vi "Multiple Rates Streaming Example.vi"() -> ()   [LabVIEW 2024]
doc: "Streaming multiple channels at different rates to a run."
uses:
  Sift API/Sift Client.lvclass
  Generate Sift Protos/SiftProxy_client/RPC Messages/sift_proxy_v1_ChannelDataType.ctl
  <vilib>/numeric/Random Number (Range) DBL.vi
  Generate Sift Protos/SiftProxy_client/SiftProxy_client.lvlib
  Sift Client.lvlib
panel:
  out "Running":bool
  out "100Hz Channel 3":dbl(knob) scale=0.0..10.0
  out "100Hz Channel 2":dbl(knob) scale=0.0..10.0
  out "100Hz Channel 1":dbl(knob) scale=0.0..10.0
  out "Loop 2 Error":errorcluster
  out "10Hz Channel 3":dbl(knob) scale=0.0..10.0
  out "10Hz Channel 2":dbl(knob) scale=0.0..10.0
  out "10Hz Channel 1":dbl(knob) scale=0.0..10.0
  out "Flush Error":errorcluster
  in  "Stop":bool
  out "Loop 1 Error":errorcluster
  in  "Organization ID":string
  in  "API Key":string
  in  "API URL":string
  # "Multiple Rates Sift Streaming Example"
  # "Instructions\n\n1. Fill in the API URL, API Key, and Organization ID. Visit this URL for more information on authentication\n    https://docs.siftstack.com/docs/api/authentication\n\n2. Start the VI\n\n3. Navigate to the Assets page and open the \"LabVIEW-Example\" asset.\n\n4. You should see the test test channels in the run.\n\n5. Click on the Live button  to see the telemetry update.\n\n6. Click Stop to stop the VI."
  # "This example streams data live from LabVIEW with channels at different rates."
  # "100Hz  Channels"
  # "These values are automatically updated randomly."
  # "Hit this to stop the example."
  # "10Hz  Channels"
  # "These values are automatically updated randomly."
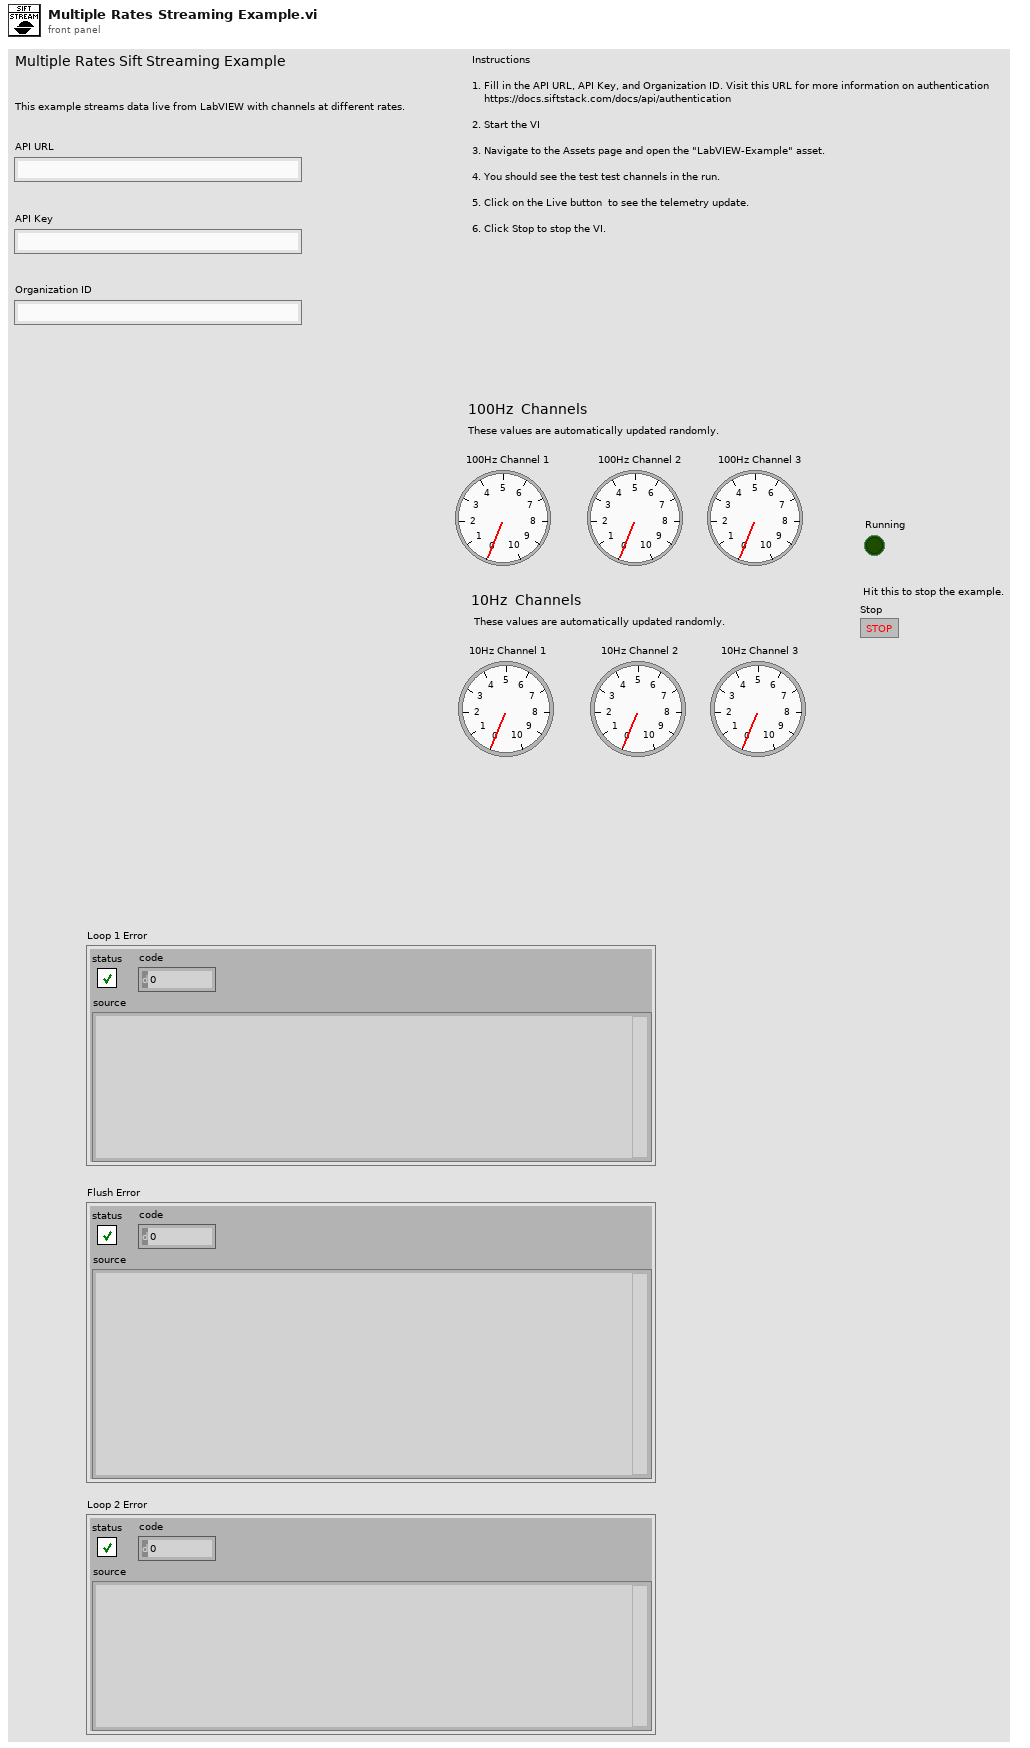
[diagram p1: front panel]
types:
  T1 = typedef "SiftProxy_client.lvlib/sift_proxy_v1_ChannelDataType.ctl" = enum32{"CHANNEL_DATA_TYPE_UNSPECIFIED", "CHANNEL_DATA_TYPE_DOUBLE", "CHANNEL_DATA_TYPE_STRING", "CHANNEL_DATA_TYPE_ENUM", "CHANNEL_DATA_TYPE_BIT_FIELD", "CHANNEL_DATA_TYPE_BOOL", "CHANNEL_DATA_TYPE_FLOAT", "CHANNEL_DATA_TYPE_INT_32", "CHANNEL_DATA_TYPE_UINT_32", "CHANNEL_DATA_TYPE_INT_64", "CHANNEL_DATA_TYPE_UINT_64"}
  T2 = typedef "SiftProxy_client.lvlib/google_protobuf_Timestamp.ctl" = cluster{"seconds":i64, "nanos":i32}
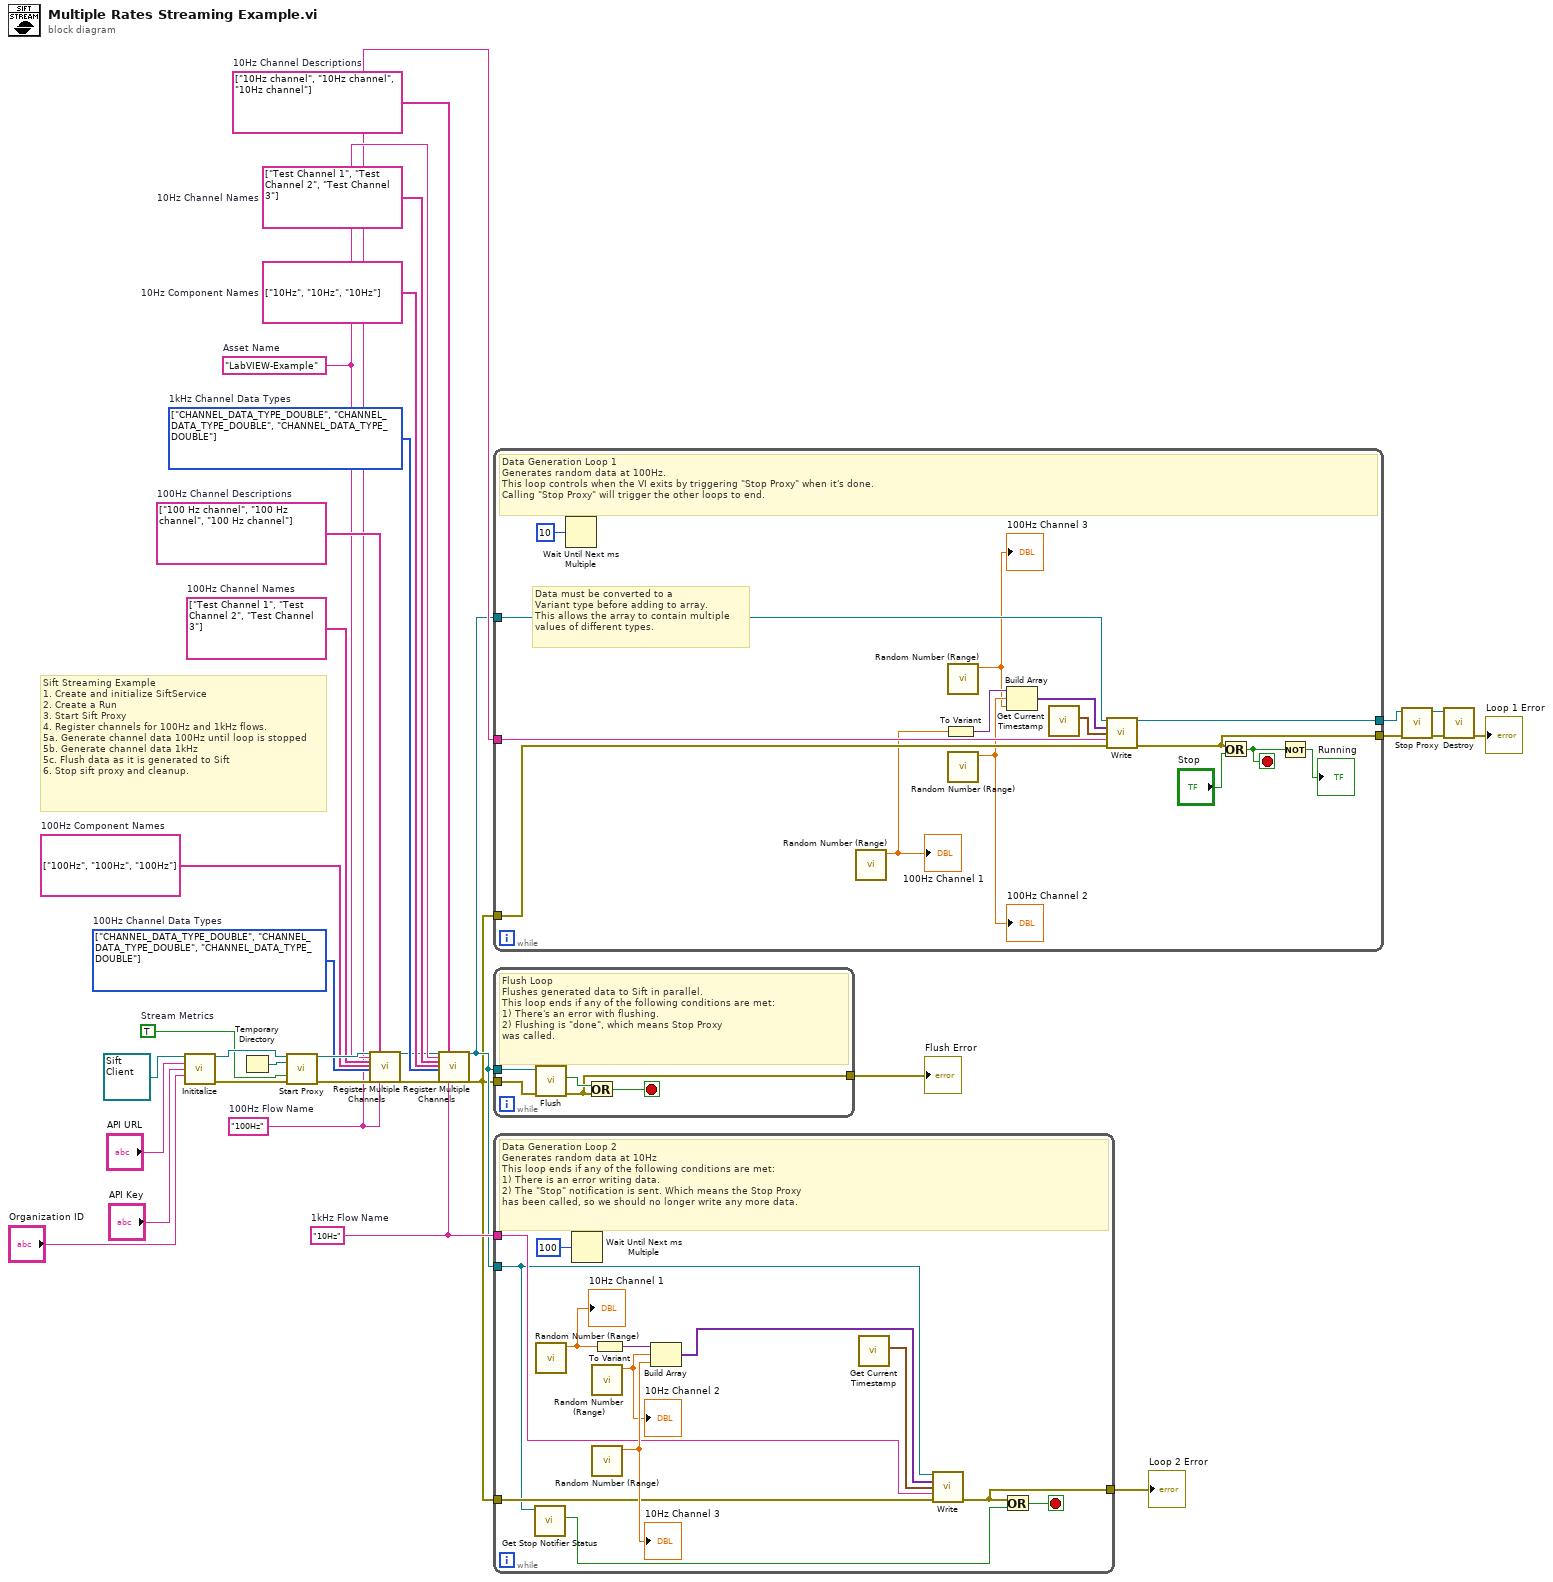
[diagram p0: block diagram]
diagram:
  w16 = string[] ["10Hz", "10Hz", "10Hz"]  # 10Hz Component Names
  w11 = "10Hz"  # 1kHz Flow Name
  w17 = string[] ["100Hz", "100Hz", "100Hz"]  # 100Hz Component Names
  w10 = "100Hz"  # 100Hz Flow Name
  w15 = T1[] [enum."CHANNEL_DATA_TYPE_DOUBLE", enum."CHANNEL_DATA_TYPE_DOUBLE", enum."CHANNEL_DATA_TYPE_DOUBLE"] items=["CHANNEL_DATA_TYPE_UNSPECIFIED", "CHANNEL_DATA_TYPE_DOUBLE", "CHANNEL_DATA_TYPE_STRING", "CHANNEL_DATA_TYPE_ENUM", "CHANNEL_DATA_TYPE_BIT_FIELD", "CHANNEL_DATA_TYPE_BOOL", "CHANNEL_DATA_TYPE_FLOAT", "CHANNEL_DATA_TYPE_INT_32", "CHANNEL_DATA_TYPE_UINT_32", "CHANNEL_DATA_TYPE_INT_64", "CHANNEL_DATA_TYPE_UINT_64"]  # 1kHz Channel Data Types
  w13 = string[] ["10Hz channel", "10Hz channel", "10Hz channel"]  # 10Hz Channel Descriptions
  w14 = string[] ["Test Channel 1", "Test Channel 2", "Test Channel 3"]  # 10Hz Channel Names
  w12 = "LabVIEW-Example"  # Asset Name
  w20 = T1[] [enum."CHANNEL_DATA_TYPE_DOUBLE", enum."CHANNEL_DATA_TYPE_DOUBLE", enum."CHANNEL_DATA_TYPE_DOUBLE"] items=["CHANNEL_DATA_TYPE_UNSPECIFIED", "CHANNEL_DATA_TYPE_DOUBLE", "CHANNEL_DATA_TYPE_STRING", "CHANNEL_DATA_TYPE_ENUM", "CHANNEL_DATA_TYPE_BIT_FIELD", "CHANNEL_DATA_TYPE_BOOL", "CHANNEL_DATA_TYPE_FLOAT", "CHANNEL_DATA_TYPE_INT_32", "CHANNEL_DATA_TYPE_UINT_32", "CHANNEL_DATA_TYPE_INT_64", "CHANNEL_DATA_TYPE_UINT_64"]  # 100Hz Channel Data Types
  w19 = string[] ["100 Hz channel", "100 Hz channel", "100 Hz channel"]  # 100Hz Channel Descriptions
  w21 = string[] ["Test Channel 1", "Test Channel 2", "Test Channel 3"]  # 100Hz Channel Names
  w26 = TRUE  # Stream Metrics
  # "Sift Streaming Example\n1. Create and initialize SiftService\n2. Create a Run\n3. Start Sift Proxy\n4. Register channels for 100Hz and 1kHz flows.\n5a. Generate channel data 100Hz until loop is stopped\n5b. Generate channel data 1kHz\n5c. Flush data as it is generated to Sift\n6. Stop sift proxy and cleanup."
  n1 = call-dynamic "Inititalize.vi"("Sift Client in"=refnum<class "Sift Client.lvclass"> refnum ("Sift Client.lvlib:Sift Client.lvclass"), "API URL"="API URL", "API Key"="API Key", "Organization ID"="Organization ID") -> ("Sift Client out"=w28:refnum<class "Sift Client.lvclass">, "error out"=w27:errorcluster)  [unwired: 10 in]
  n2 = Temporary Directory() -> (w1:path)
  n3 = call-dynamic "Start Proxy.vi"("Sift Client in"=w28, "Storage Path"=w1, "Stream Metrics"=w26, "error in (no error)"=w27) -> ("Sift Client out"=w22:refnum<class "Sift Client.lvclass">, "error out"=w23:errorcluster)  [unwired: 10 in]
  n4 = call "Register Multiple Channels.vi"("Sift Client in"=w22, "Asset Name"=w12, "Names"=w21, "Components"=w17, "Data Types"=w20, "error in (no error)"=w23, "Descriptions"=w19, "Flow Name"=w10) -> ("Sift Client out"=w9:refnum<class "Sift Client.lvclass">, "error out"=w7:errorcluster)  [unwired: 18 in]
  n5 = call "Register Multiple Channels.vi"("Sift Client in"=w9, "Asset Name"=w12, "Names"=w14, "Components"=w16, "Data Types"=w15, "error in (no error)"=w7, "Descriptions"=w13, "Flow Name"=w11) -> ("Sift Client out"=w8:refnum<class "Sift Client.lvclass">, "error out"=w6:errorcluster)  [unwired: 18 in]
  n6 = while {
    tunnel: w8 -> [w47]
    tunnel: w6 -> [w46]
    tunnel: [w41] -> w18
    tunnel: [w42] -> w3
    tunnel: w10 -> [w39]
    stop <- w33 stop-if-true
    # "Data must be converted to a \nVariant type before adding to array.\nThis allows the array to contain multiple \nvalues of different types."
    # "Data Generation Loop 1\nGenerates random data at 100Hz.\nThis loop controls when the VI exits by triggering \"Stop Proxy\" when it's done. \nCalling \"Stop Proxy\" will trigger the other loops to end."
    n7 = Wait Until Next ms Multiple(millisecond multiple=u32 10 ("milliseconds to wait")) -> ()  [unwired: 1 out]
    n8 = call-poly <vilib>:"Random Number (Range).vi"() -> ("number"=w36:dbl)  [unwired: 11 in]
    "100Hz Channel 1" <- w36
    n9 = To Variant(anything=w36) -> (Variant=w45:variant)
    n10 = call-poly <vilib>:"Random Number (Range).vi"() -> ("number"=w37:dbl)  [unwired: 11 in]
    "100Hz Channel 3" <- w37
    n11 = call-poly <vilib>:"Random Number (Range).vi"() -> ("number"=w38:dbl)  [unwired: 11 in]
    "100Hz Channel 2" <- w38
    n12 = Build Array(w45, w38, w37) -> (w44:variant[])
    n13 = call "Get Current Timestamp.vi"() -> ("Timestamp"=w43:T2)  [unwired: 11 in]
    n14 = call-dynamic "Write.vi"("Sift Client in"=w47, "Values"=w44, "Timestamp"=w43, "Flow Name"=w39, "error in (no error)"=w46) -> ("Sift Client out"=w41:refnum<class "Sift Client.lvclass">, "error out"=w42:errorcluster)  [unwired: 9 in]
    n15 = Or(x=w42, y="Stop") -> (x .or. y?=w33:bool)
    n16 = Not(x=w33) -> (.not. x?=→"Running":bool)
  }
  n17 = while {
    tunnel: w8 -> [w52]
    tunnel: w6 -> [w51]
    tunnel: [w49] -> w4
    stop <- w48 stop-if-true
    # "Flush Loop\nFlushes generated data to Sift in parallel.\nThis loop ends if any of the following conditions are met:\n1) There's an error with flushing.\n2) Flushing is \"done\", which means Stop Proxy \nwas called."
    n18 = call-dynamic "Flush.vi"("error in (no error)"=w51, "Sift Client in"=w52) -> ("error out"=w49:errorcluster, "Done"=w50:bool)  [unwired: 7 in, 1 out]
    n19 = Or(x=w50, y=w49) -> (x .or. y?=w48:bool)
  }
  "Flush Error" <- w4
  n20 = while {
    tunnel: w11 -> [w59]
    tunnel: w8 -> [w55]
    tunnel: w6 -> [w58]
    tunnel: [w57] -> w5
    stop <- w56 stop-if-true
    # "Data Generation Loop 2\nGenerates random data at 10Hz\nThis loop ends if any of the following conditions are met:\n1) There is an error writing data.\n2) The \"Stop\" notification is sent. Which means the Stop Proxy \nhas been called, so we should no longer write any more data."
    n21 = call-dynamic "Get Stop Notifier Status.vi"("Sift Client in"=w55) -> ("Fired"=w54:bool)  [unwired: 8 in, 2 out]
    n22 = call-poly <vilib>:"Random Number (Range).vi"() -> ("number"=w63:dbl)  [unwired: 11 in]
    "10Hz Channel 1" <- w63
    n23 = Wait Until Next ms Multiple(millisecond multiple=u32 100 ("milliseconds to wait")) -> ()  [unwired: 1 out]
    n24 = call-poly <vilib>:"Random Number (Range).vi"() -> ("number"=w64:dbl)  [unwired: 11 in]
    "10Hz Channel 2" <- w64
    n25 = call-poly <vilib>:"Random Number (Range).vi"() -> ("number"=w65:dbl)  [unwired: 11 in]
    "10Hz Channel 3" <- w65
    n26 = To Variant(anything=w63) -> (Variant=w62:variant)
    n27 = Build Array(w62, w64, w65) -> (w61:variant[])
    n28 = call "Get Current Timestamp.vi"() -> ("Timestamp"=w60:T2)  [unwired: 11 in]
    n29 = call-dynamic "Write.vi"("Sift Client in"=w55, "Values"=w61, "Timestamp"=w60, "Flow Name"=w59, "error in (no error)"=w58) -> ("error out"=w57:errorcluster)  [unwired: 9 in, 1 out]
    n30 = Or(x=w57, y=w54) -> (x .or. y?=w56:bool)
  }
  "Loop 2 Error" <- w5
  n31 = call-dynamic "Stop Proxy.vi"("error in (no error)"=w3, "Sift Client in"=w18) -> ("error out"=w2:errorcluster, "Sift Client out"=w25:refnum<class "Sift Client.lvclass">)  [unwired: 7 in, 1 out]
  n32 = call-dynamic "Destroy.vi"("error in (no error)"=w2, "Sift Client in"=w25) -> ("error out"=→"Loop 1 Error":errorcluster)  [unwired: 8 in, 1 out]
